vi "DFD FXP Get Quantizer.vi"   [LabVIEW 2017, in "NI_DigFilterLicensed.lvlib"]
doc: "Retrieves quantizer settings from a fixed-point filter. You must manually select the polymorphic instance you want to use."
uses:
  <vilib>/addons/Digital Filter Design/NI_DigFilterLicensed.lvlib
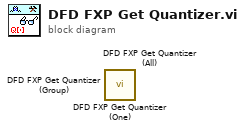
[diagram p0: block diagram]
diagram:
  n1 = call <vilib>:"DFD FXP Get Quantizer (One).vi"() -> ()  [unwired: 9 in, 3 out]
  n2 = call <vilib>:"DFD FXP Get Quantizer (All).vi"() -> ()  [unwired: 9 in, 3 out]
  n3 = call <vilib>:"DFD FXP Get Quantizer (Group).vi"() -> ()  [unwired: 9 in, 3 out]
